vi "Pre-Build VI - Run Unit Tests.vi"(8 "error in (no error)":errorcluster) -> (0 "error out":errorcluster, 1 "VIs without test coverage":string[](array[string]), 2 "error type":enum16{"fatal", "non-fatal", "warning"}(ring), 4 "VIs not loadable":string[](array[string]))   [LabVIEW 2009]
uses:
  <userlib>/_OpenG.lib/array/array.llb/Conditional Auto-Indexing Tunnel (String)__ogtk.vi
  <userlib>/_OpenG.lib/array/array.llb/Empty 1D Array (String)__ogtk.vi
  <userlib>/_OpenG.lib/array/array.llb/Filter 1D Array (String)__ogtk.vi
panel:
  out "VIs Failed":string[](array[string])
  out "VIs Succeeded":string[](array[string])
  in  "type specifier VI Refnum (for type only)":refnum<vi>
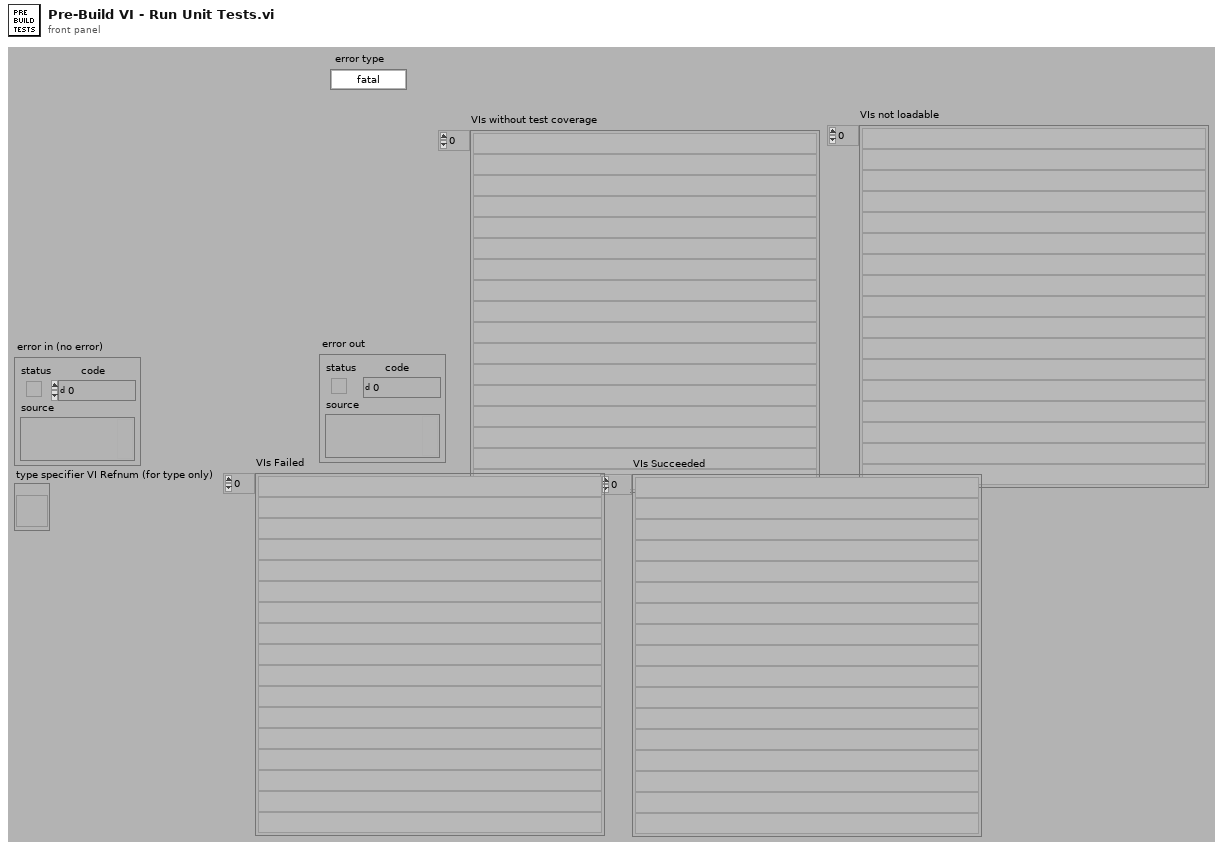
[diagram p1: front panel]
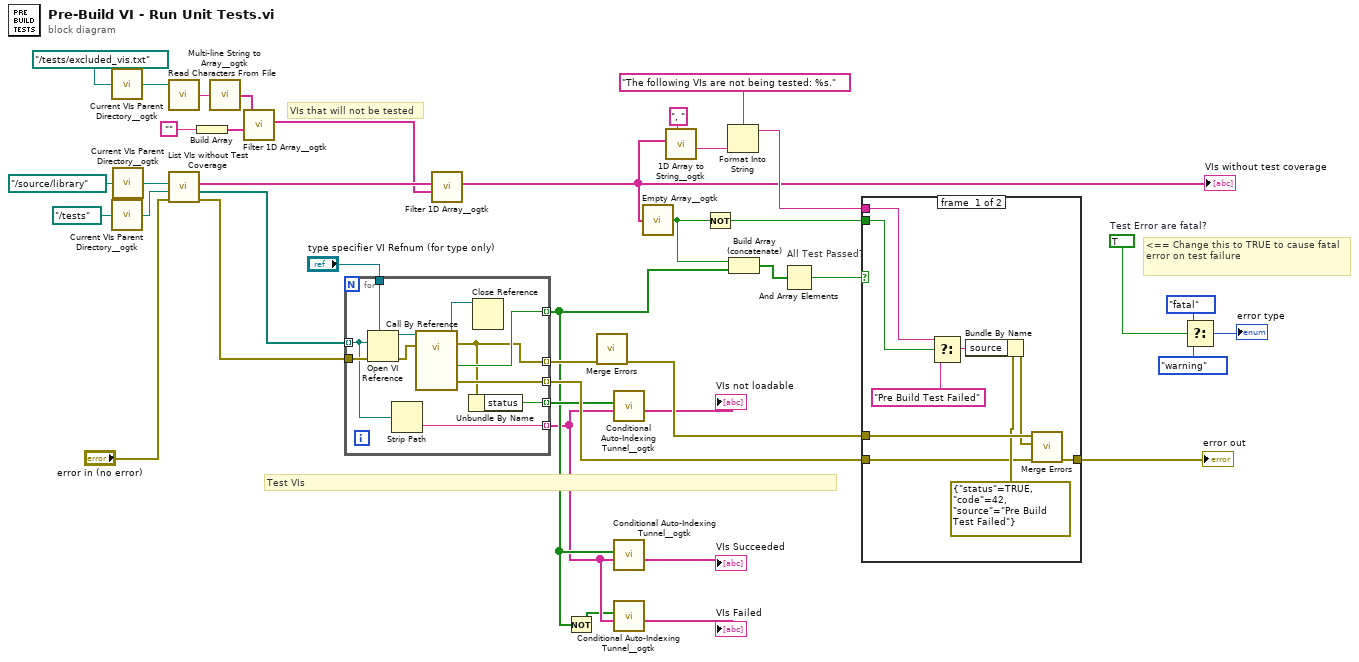
[diagram p0: block diagram]
diagram:
  w27 = TRUE  # Test Error are fatal?
  # "VIs that will not be tested"
  # "<== Change this to TRUE to cause fatal error on test failure"
  # "All Test Passed?"
  # "Test VIs"
  n1 = call <userlib>:"Current VIs Parent Directory__ogtk.vi"("Relative path (.)"=path "../tests/excluded_vis.txt") -> ("Parent Directory (+ Relative)"=w16:path)  [unwired: 4 in]
  n2 = call <userlib>:"Current VIs Parent Directory__ogtk.vi"("Relative path (.)"=path "../tests") -> ("Parent Directory (+ Relative)"=w21:path)  [unwired: 4 in]
  n3 = call <userlib>:"Current VIs Parent Directory__ogtk.vi"("Relative path (.)"=path "../source/library") -> ("Parent Directory (+ Relative)"=w31:path)  [unwired: 4 in]
  n4 = call <vilib>:"Read Characters From File.vi"("file path (dialog if empty)"=w16) -> ("character string"=w15:string)  [unwired: 5 in, 3 out]
  n5 = call "List VIs without Test Coverage.vi"("error in (no error)"="error in (no error)", "Tests Root"=w21, "Source Root"=w31) -> ("error out"=w10:errorcluster, "Test VIs"=w20:path[], "VIs without test coverage"=w38:string[])  [unwired: 6 in]
  n6 = Build Array("") -> (w12:string[])
  n7 = call <userlib>:"Multi-line String to Array__ogtk.vi"("string"=w15) -> ("lines"=w14:string[])
  n8 = call-poly <userlib>:"Filter 1D Array__ogtk.vi"("items to filter"=w12, "array"=w14) -> ("filtered array"=w11:string[])  [unwired: 4 in, 1 out]
  n9 = for {
    tunnel: w20 -> [w42] mode=indexing
    tunnel: "type specifier VI Refnum (for type only)" -> [w51]
    tunnel: [w48] -> w4 mode=indexing
    tunnel: [w46] -> w18 mode=indexing
    tunnel: w10 -> [w45]
    tunnel: [w44] -> w8 mode=indexing
    tunnel: [w43] -> w5 mode=indexing
    tunnel: [w41] -> w2 mode=indexing
    n10 = Open VI Reference(type specifier VI Refnum (for type only)=w51, vi path=w42, error in (no error)=w45) -> (vi reference=w50:refnum<vi>, error out=w49:errorcluster)  [unwired: 3 in]
    n11 = Strip Path(path=w42) -> (name=w41:string)  [unwired: 1 out]
    n12 = call-by-ref "?"(reference=w50, error in=w49) -> (reference out=w47:refnum<vi>, error out=w44:errorcluster, 0:"error out"=w46:errorcluster, "pass"=w48:bool)  [unwired: 10 in]
    n13 = Unbundle By Name(w44) -> ("status"=w43:bool)
    n14 = Close Reference(reference=w47) -> ()  [unwired: 1 in, 1 out]
  }
  n15 = call-poly <userlib>:"Filter 1D Array__ogtk.vi"("items to filter"=w11, "array"=w38) -> ("filtered array"=w23:string[])  [unwired: 4 in, 1 out]
  "VIs without test coverage" <- w23
  n16 = Not(x=w4) -> (.not. x?=w1:bool[])
  n17 = call <vilib>:"Merge Errors.vi"("error array in"=w8) -> ("error out"=w9:errorcluster)  [unwired: 6 in]
  n18 = call-poly <userlib>:"Conditional Auto-Indexing Tunnel__ogtk.vi"("Array in"=w2, "Elements to keep"=w5) -> ("Filtered Array out"=→"VIs not loadable":string[])  [unwired: 5 in]
  n19 = call-poly <userlib>:"Conditional Auto-Indexing Tunnel__ogtk.vi"("Array in"=w2, "Elements to keep"=w4) -> ("Filtered Array out"=→"VIs Succeeded":string[])  [unwired: 5 in]
  n20 = call-poly <userlib>:"Conditional Auto-Indexing Tunnel__ogtk.vi"("Array in"=w2, "Elements to keep"=w1) -> ("Filtered Array out"=→"VIs Failed":string[])  [unwired: 5 in]
  n21 = call-poly <userlib>:"Empty Array__ogtk.vi"("Array"=w23) -> ("Empty Array?"=w33:bool)  [unwired: 8 in]
  n22 = call <userlib>:"1D Array to String__ogtk.vi"("delimiter (Tab)"=", ", "Array of Strings"=w23) -> ("delimited string"=w36:string)  [unwired: 9 in]
  n23 = Not(x=w33) -> (.not. x?=w32:bool)
  n24 = Format Into String(format string="The following VIs are not being tested: %s.", w36) -> (resulting string=w34:string)  [unwired: 2 in, 1 out]
  n25 = Build Array (concatenate)(w33, w4) -> (w40:bool[])
  n26 = And Array Elements(Boolean array=w40) -> (logical AND=w39:bool)
  n27 = case shown="False" w39 {
    tunnel: w9 -> [w60 w61]
    tunnel: [w59 w61] -> w29
    tunnel: w32 -> [w58 _]
    tunnel: w34 -> [w57 _]
    tunnel: w18 -> [w52 _]
    frame #0 {
      n28 = Select(t=w57, s=w58, f="Pre Build Test Failed" ("source")) -> (s? t:f=w55:string)
      n29 = Bundle By Name(cluster=errorcluster {"status"=TRUE, "code"=42, "source"="Pre Build Test Failed"} ("error out"), "source"=w55) -> (w54:errorcluster)
      n30 = call <vilib>:"Merge Errors.vi"("error array in"=w52, "error in 2 (no error)"=w54, "error in 1 (no error)"=w60) -> ("error out"=w59:errorcluster)  [unwired: 4 in]
    }
    frame #1 {
    }
  }
  "error out" <- w29
  n31 = Select(t=enum16{"fatal", "non-fatal", "warning"}."fatal" ("error type"), s=w27, f=enum16{"fatal", "non-fatal", "warning"}."warning" ("error type")) -> (s? t:f=→"error type":enum16{"fatal", "non-fatal", "warning"})
